vi "insert_missing_peak.vi"(6 "Approximate Phase Difference":dbl, 8 "missing peak index in":i32, 9 "Phase in":dbl[](array[numeric]), 10 "Boolean":bool, 11 "Numeric":i32) -> (0 "missing peak index out":i32, 3 "Phase out":dbl[](array[numeric]))   [LabVIEW 2016]
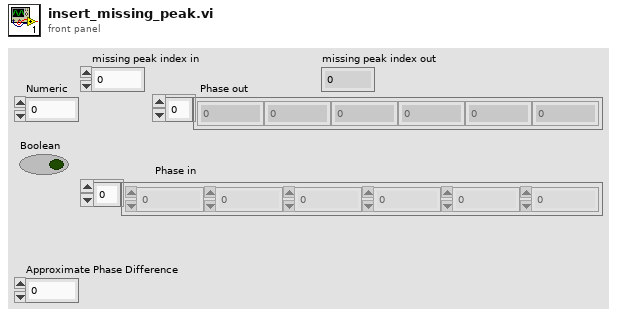
[diagram p1: front panel]
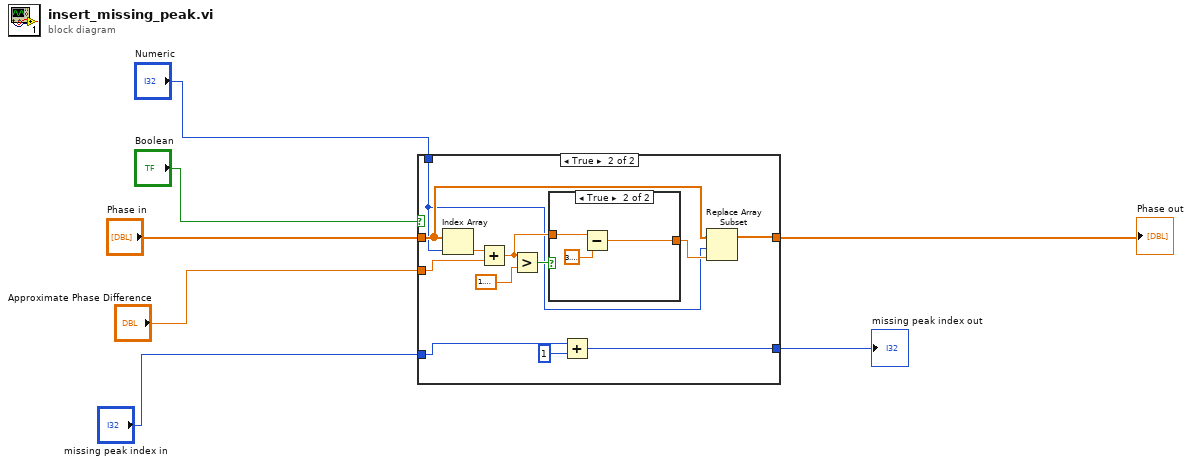
[diagram p0: block diagram]
diagram:
  n1 = case shown="True" "Boolean" {
    tunnel: "Phase in" -> [w9 w16]
    tunnel: [w9 w15] -> w4
    tunnel: "Approximate Phase Difference" -> [_ w20]
    tunnel: "Numeric" -> [_ w10]
    tunnel: "missing peak index in" -> [w8 w14]
    tunnel: [w8 w12] -> w1
    frame False {
    }
    frame True {
      n2 = Index Array(array=w16, index=w10) -> (element=w21:dbl)
      n3 = Add(x=w21, y=w20) -> (x+y=w17:dbl)
      n4 = Greater?(x=w17, y=1.5707963267948966) -> (0:w19:bool)
      n5 = case shown="True" w19 {
        tunnel: w17 -> [w22 w25]
        tunnel: [w22 w23] -> w11
        frame False {
        }
        frame True {
          n6 = Subtract(x=w25, y=3.141592653589793) -> (x-y=w23:dbl)
        }
      }
      n7 = Add(x=w14, y=1) -> (x+y=w12:i32)
      n8 = Replace Array Subset(array=w16, new element=w11, index=w10) -> (w15:dbl[])
    }
  }
  "Phase out" <- w4
  "missing peak index out" <- w1
